vi "main 6th.vi"() -> ()   [LabVIEW 2015]
panel:
  out "6":u32
  out "3":u32
  out "1":u32
  out "2":u32
  out "5":u32
  out "4":u32
  in  "dimension size 2":i32
  in  "dimension size":i32
  out "Array":u16[][](array[numeric])
  out "element":u16[][](array[numeric])
  out "From OD fit?":bool
  in  "Current file num":i32
  in  "Fitting Results Save Path":string[](array[string])
  in  "Initial guess values":dbl[](array[numeric])
  out "Latest image data":dbl[][](array[numeric])
  in  "Fitting Type":u16(ring)
  in  "Force Guess?":bool
  in  "milliseconds to wait":u32
  out "best fit parameters":dbl[](array[numeric])
  in  "Reset process index":bool
  out "ROI Height":u32
  out "ROI Width":u32
  out "OD image":u16[][](graph)
  out "Process Index":i32
  out "External Trigger":bool
  out "XY图":cluster{i32[], dbl[]}[](graph)
  in  "OD fit":bool
  in  "OD num":i32
  out "Fit Done":bool
  in  "Exit":bool
  out "XY图 2":cluster{i32[], dbl[]}[](graph)
  in  "Fit":bool
  in  "Open File":bool
  in  "Auto Fit":bool
  in  "Stop":bool
  in  "Aquire":bool
  in  "Fitting Config":bool
  in  "Camera Config":bool
  in  "Initialize":bool
  in  "Live Image Display":refnum<k7>(container)
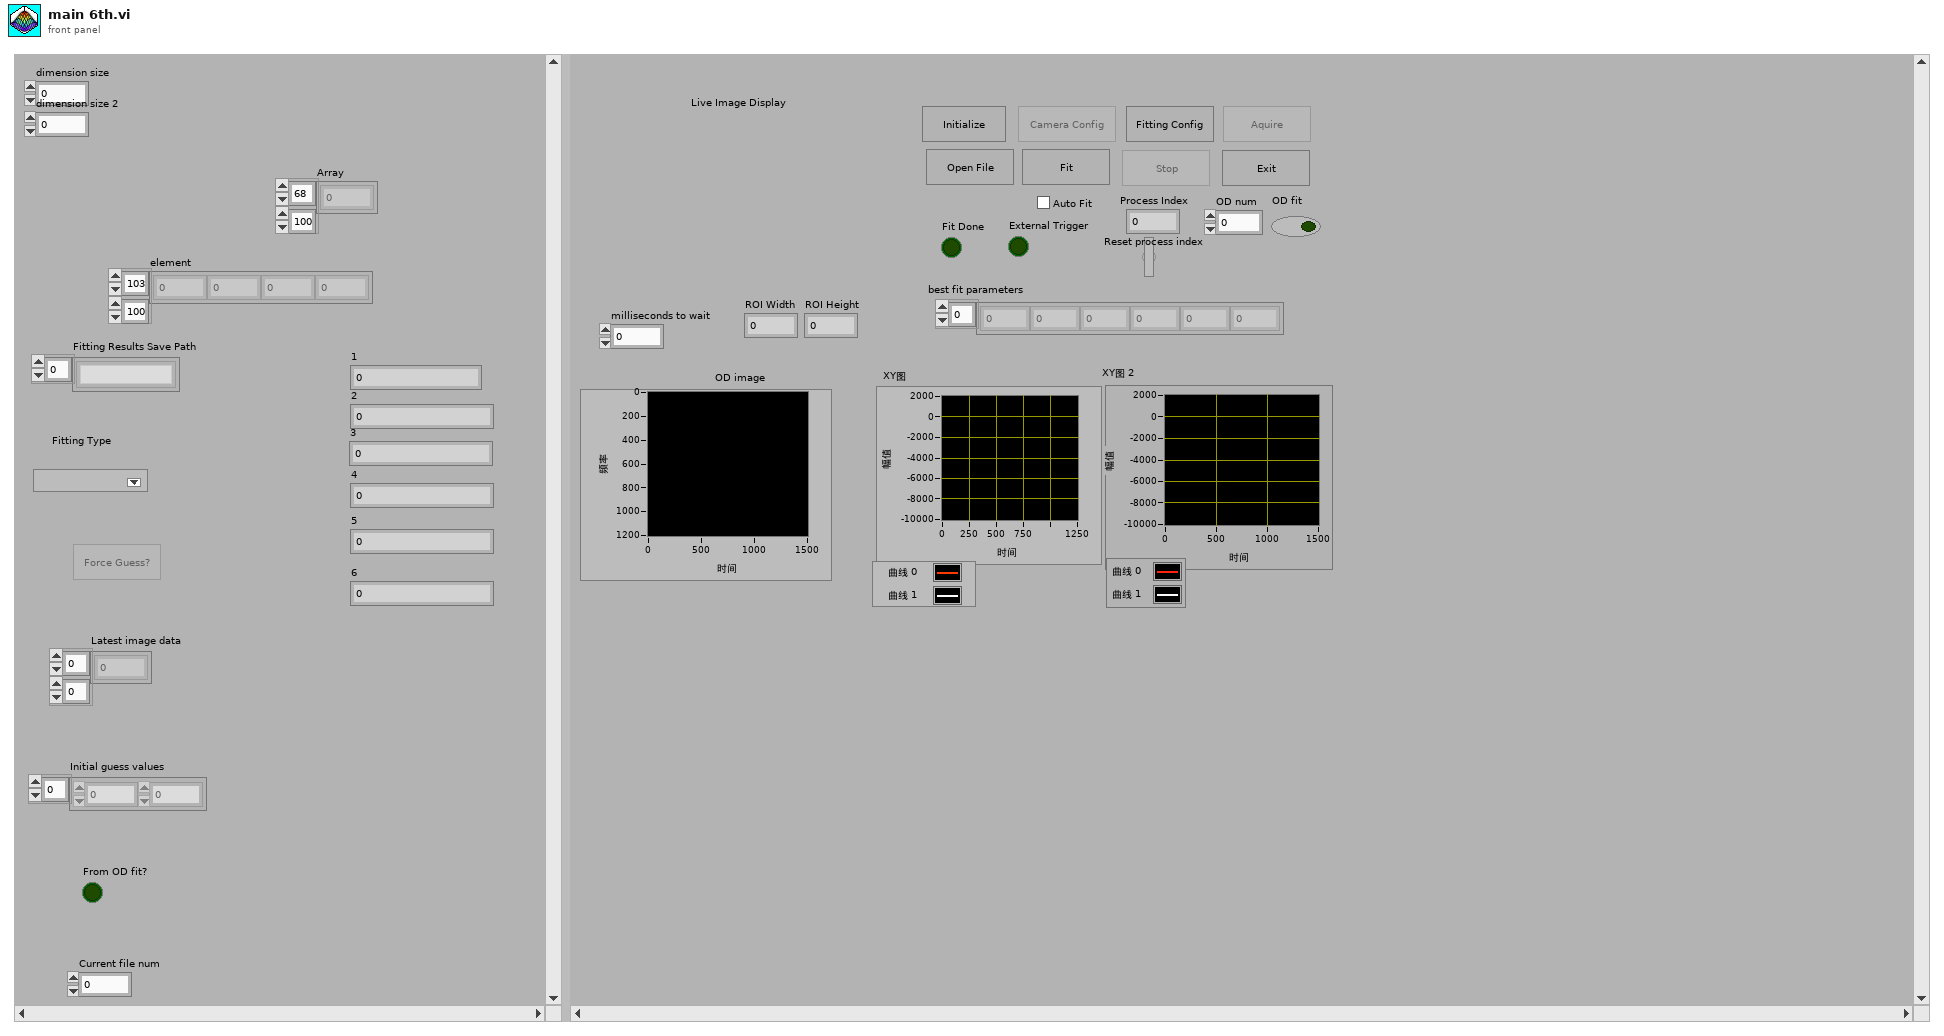
[diagram p1: front panel]
types:
  T1 = enum8{"Enabled", "Disabled", "Disabled and Grayed Out"}
  T2 = typedef "Image Type" = u32
  T3 = typedef "IMAQ Image.ctl" = refnum<image>
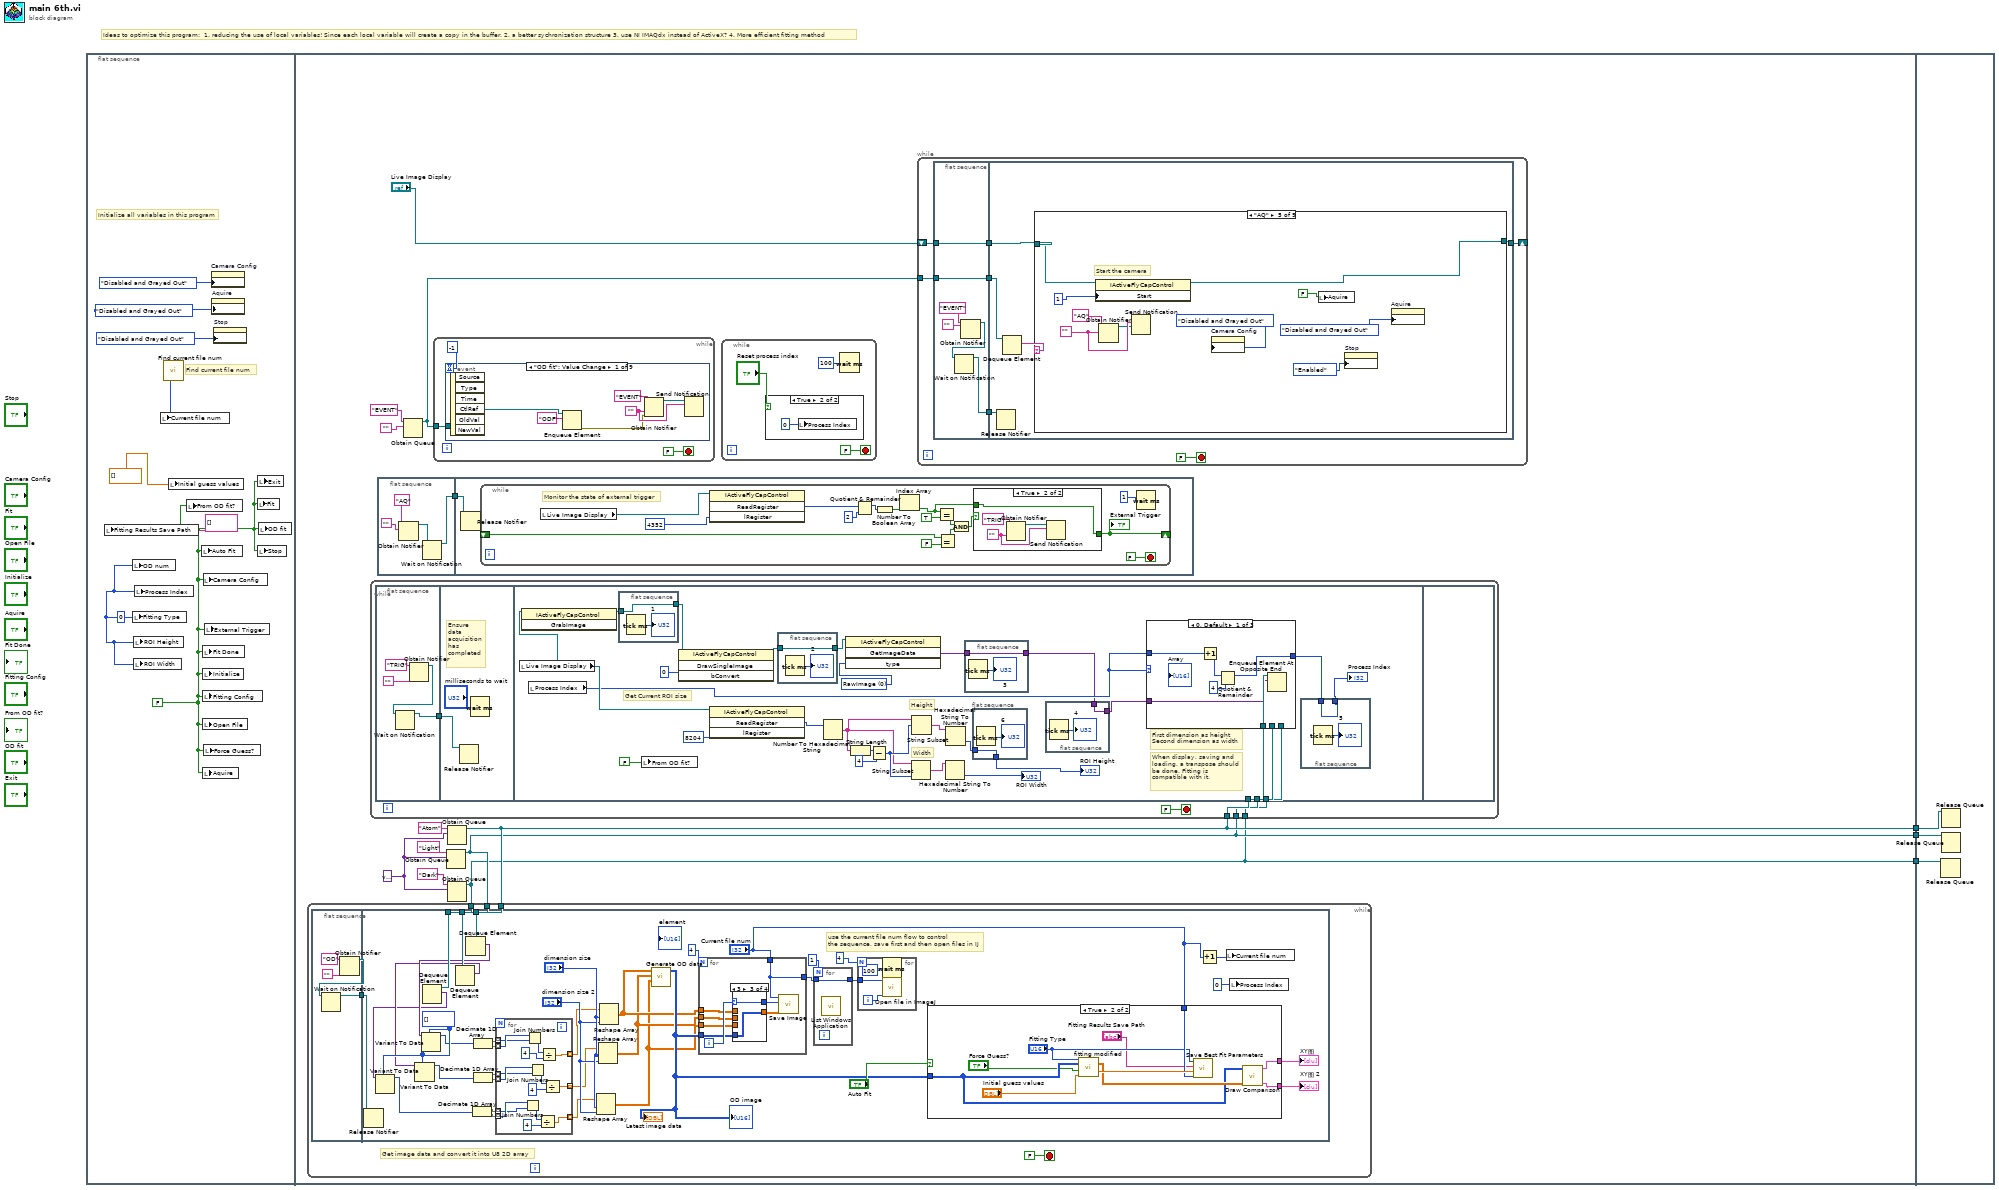
[diagram p0: block diagram]
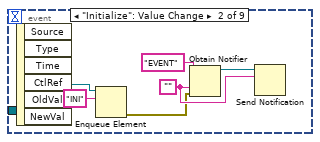
[diagram p2: hidden frame]
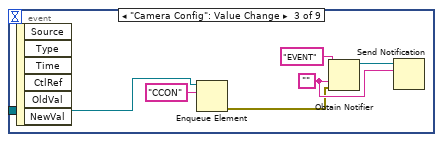
[diagram p3: hidden frame]
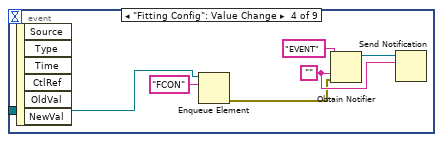
[diagram p4: hidden frame]
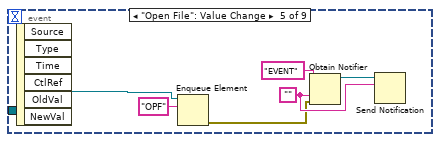
[diagram p5: hidden frame]
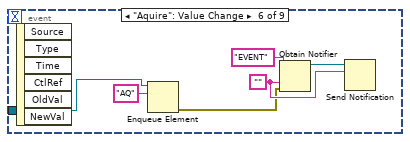
[diagram p6: hidden frame]
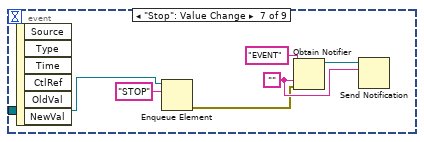
[diagram p7: hidden frame]
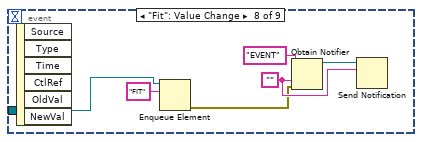
[diagram p8: hidden frame]
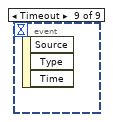
[diagram p9: hidden frame]
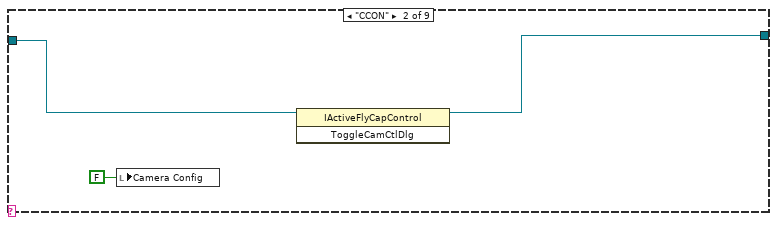
[diagram p11: hidden frame]
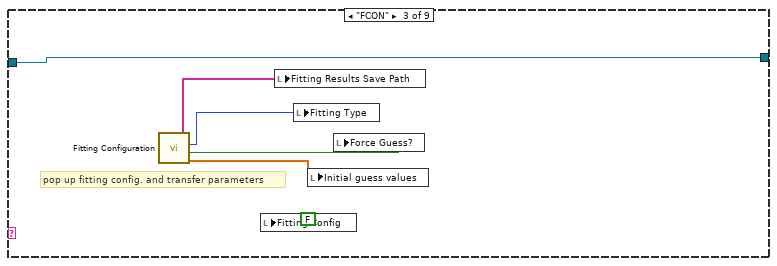
[diagram p12: hidden frame]
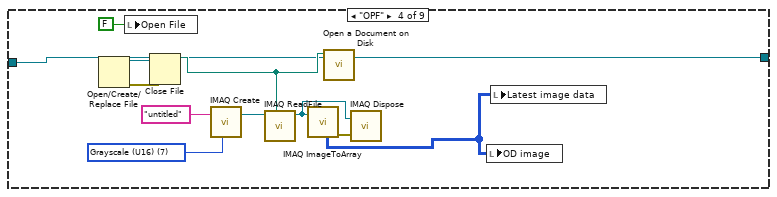
[diagram p13: hidden frame]
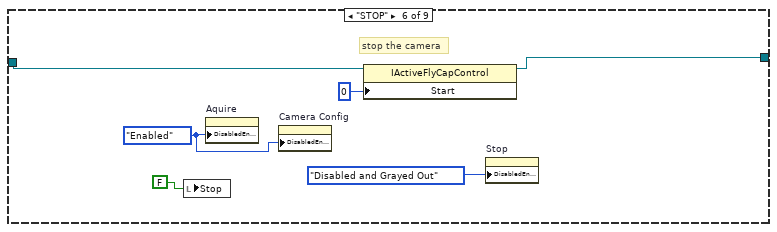
[diagram p14: hidden frame]
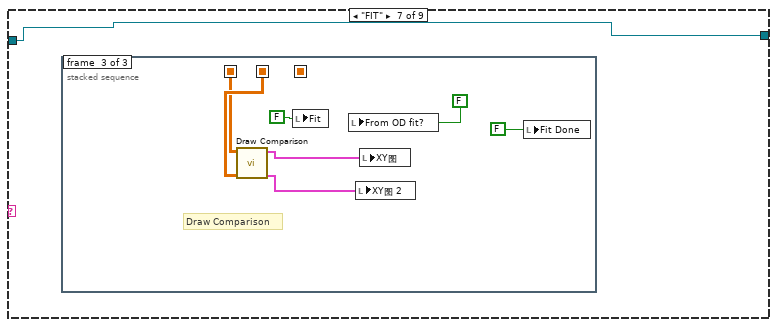
[diagram p15: hidden frame]
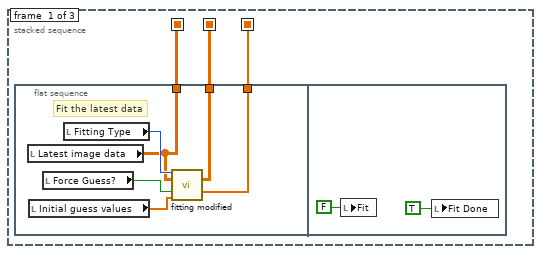
[diagram p16: hidden frame]
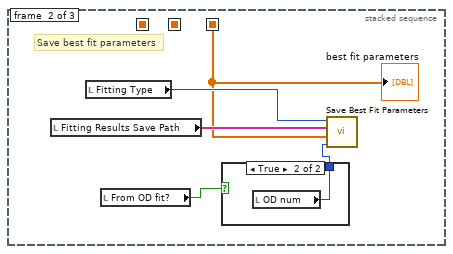
[diagram p17: hidden frame]
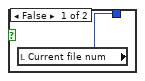
[diagram p18: hidden frame]
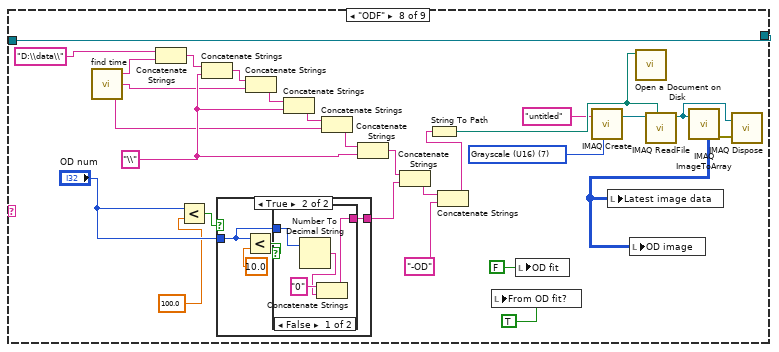
[diagram p19: hidden frame]
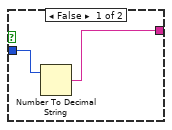
[diagram p20: hidden frame]
diagram:
  # "Ideas to optimize this program:  1. reducing the use of local variables! Since each local variable will create a copy in the buffer. 2. a better sychronization structure 3. use NI IMAQdx instead of ActiveX? 4. More efficient fitting method"
  n1 = flat-sequence {
    tunnel: [w19] -> w3
    tunnel: [w18] -> w2
    tunnel: [w17] -> w1
    tunnel: w3 -> [w411]
    tunnel: w2 -> [w410]
    tunnel: w1 -> [w409]
    frame #0 {
      w7 = 0 ("OD num")
      w5 = FALSE ("Aquire")
      # "Find current file num"
      # "Initialize all variables in this program"
      n2 = local write "Fitting Results Save Path"(string[] [] ("Fitting Results Save Path")) -> ()
      n3 = local write "OD num"(w7) -> ()
      n4 = local write "Fitting Type"(w7) -> ()
      n5 = local write "ROI Height"(w7) -> ()
      n6 = local write "ROI Width"(w7) -> ()
      n7 = local write "Process Index"(w7) -> ()
      n8 = call "Find current file num.vi"() -> ("Current File Num"=w4:u16)  [unwired: 2 in]
      n9 = local write "Current file num"(w4) -> ()
      n10 = local write "Initial guess values"(dbl[] [] ("Best fit parameters")) -> ()
      n11 = local write "From OD fit?"(w5) -> ()
      n12 = local write "Auto Fit"(w5) -> ()
      n13 = local write "Fit Done"(w5) -> ()
      n14 = local write "Initialize"(w5) -> ()
      n15 = local write "Fitting Config"(w5) -> ()
      n16 = local write "Open File"(w5) -> ()
      n17 = local write "Aquire"(w5) -> ()
      n18 = local write "Camera Config"(w5) -> ()
      n19 = local write "Force Guess?"(w5) -> ()
      n20 = local write "External Trigger"(w5) -> ()
      n21 = property on="Camera Config" class="Bool (strict)"("DisabledEnum"=T1."Disabled and Grayed Out" ("禁用")) -> ()  [unwired: 2 in, 2 out]
      n22 = property on="Aquire" class="Bool (strict)"("DisabledEnum"=T1."Disabled and Grayed Out" ("禁用")) -> ()  [unwired: 2 in, 2 out]
      n23 = property on="Stop" class="Bool (strict)"("DisabledEnum"=T1."Disabled and Grayed Out" ("禁用")) -> ()  [unwired: 2 in, 2 out]
      n24 = local write "Fit"(w5) -> ()
      n25 = local write "Exit"(w5) -> ()
      n26 = local write "Stop"(w5) -> ()
      n27 = local write "OD fit"(w5) -> ()
    }
    frame #1 {
      w13 = variant
      n28 = flat-sequence {
        tunnel: [w307] -> w23
        tunnel: w23 -> [w311]
        frame #0 {
          n29 = Obtain Notifier(name (unnamed)="AQ" ("名称（未命名）"), notification data type="") -> (notifier out=w309:refnum<notifier>)  [unwired: 2 in, 2 out]
          n30 = Wait on Notification(notifier=w309) -> (notifier out=w307:refnum<notifier>)  [unwired: 3 in, 3 out]
        }
        frame #1 {
          n31 = Release Notifier(notifier=w311) -> ()  [unwired: 2 in, 3 out]
          n32 = while {
            shift-right: [w314] -> _
            shift-left: _ -> [w313]
            stop <- FALSE stop-if-true
            # "Monitor the state of external trigger"
            n33 = local read "Live Image Display"() -> (w327:refnum<k7>)
            n34 = invoke class="IActiveFlyCapControl" method="ReadRegister"(reference=w327, "lRegister"=u32 4352) -> ("ReadRegister"=w325:u32)  [unwired: 2 in, 3 out]
            n35 = Quotient & Remainder(x=w325, y=u32 2) -> (x-y*floor(x/y)=w323:u32)  [unwired: 1 out]
            n36 = Number To Boolean Array(number=w323) -> (Boolean array=w322:bool[])
            n37 = Index Array(array=w322) -> (element=w316:bool)  [unwired: 1 in]
            n38 = Equal?(x=w316, y=TRUE) -> (x = y?=w318:bool)
            n39 = Equal?(x=w313, y=FALSE) -> (x = y?=w319:bool)
            n40 = And(x=w318, y=w319) -> (x .and. y?=w317:bool)
            n41 = case shown="True" w317 {
              tunnel: w316 -> [w328 w329]
              tunnel: [w328 w329] -> w314
              frame False {
              }
              frame True {
                w330 = ""
                n42 = Obtain Notifier(name (unnamed)="TRIG" ("名称（未命名）"), notification data type=w330) -> (notifier out=w331:refnum<notifier>)  [unwired: 2 in, 2 out]
                n43 = Send Notification(notification=w330, notifier=w331) -> ()  [unwired: 1 in, 2 out]
              }
            }
            "External Trigger" <- w314
            n44 = Wait (ms)(milliseconds to wait=u32 1) -> ()  [unwired: 1 out]
          }
        }
      }
      n45 = Obtain Queue(name (unnamed)="EVENT" ("名称（未命名）"), element data type="") -> (queue out=w14:refnum<queue>)  [unwired: 3 in, 2 out]
      n46 = while {
        tunnel: w14 -> [w24]
        stop <- FALSE stop-if-true
        n47 = event shown="[0] \"OD fit\": Value Change" {
          selector: _ -> [_ _ _ _ _ _ _ _ _]
          dyn-events: _ -> [_ _ _ _ _ _ _ _ _]
          timeout: -1 -> [_ _ _ _ _ _ _ _ _]
          tunnel: w24 -> [w27 w34 w39 w45 w51 w57 w63 w69 _]
          event "OD fit": Value Change {
            w30 = ""
            n48 = event-data() -> ()  [unwired: 1 in, 6 out]
            n49 = Enqueue Element(queue=w27, element="ODF") -> (error out=w28:errorcluster)  [unwired: 2 in, 2 out]
            n50 = Obtain Notifier(name (unnamed)="EVENT" ("名称（未命名）"), notification data type=w30, error in (no error)=w28) -> (notifier out=w31:refnum<notifier>)  [unwired: 1 in, 2 out]
            n51 = Send Notification(notification=w30, notifier=w31) -> ()  [unwired: 1 in, 2 out]
          }
          event "Initialize": Value Change {
            w36 = ""
            n52 = event-data() -> ()  [unwired: 1 in, 6 out]
            n53 = Enqueue Element(queue=w34, element="INI") -> (error out=w33:errorcluster)  [unwired: 2 in, 2 out]
            n54 = Obtain Notifier(name (unnamed)="EVENT" ("名称（未命名）"), notification data type=w36, error in (no error)=w33) -> (notifier out=w37:refnum<notifier>)  [unwired: 1 in, 2 out]
            n55 = Send Notification(notification=w36, notifier=w37) -> ()  [unwired: 1 in, 2 out]
          }
          event "Camera Config": Value Change {
            w42 = ""
            n56 = event-data() -> ()  [unwired: 1 in, 6 out]
            n57 = Enqueue Element(queue=w39, element="CCON") -> (error out=w40:errorcluster)  [unwired: 2 in, 2 out]
            n58 = Obtain Notifier(name (unnamed)="EVENT" ("名称（未命名）"), notification data type=w42, error in (no error)=w40) -> (notifier out=w43:refnum<notifier>)  [unwired: 1 in, 2 out]
            n59 = Send Notification(notification=w42, notifier=w43) -> ()  [unwired: 1 in, 2 out]
          }
          event "Fitting Config": Value Change {
            w48 = ""
            n60 = event-data() -> ()  [unwired: 1 in, 6 out]
            n61 = Enqueue Element(queue=w45, element="FCON") -> (error out=w46:errorcluster)  [unwired: 2 in, 2 out]
            n62 = Obtain Notifier(name (unnamed)="EVENT" ("名称（未命名）"), notification data type=w48, error in (no error)=w46) -> (notifier out=w49:refnum<notifier>)  [unwired: 1 in, 2 out]
            n63 = Send Notification(notification=w48, notifier=w49) -> ()  [unwired: 1 in, 2 out]
          }
          event "Open File": Value Change {
            w54 = ""
            n64 = event-data() -> ()  [unwired: 1 in, 6 out]
            n65 = Enqueue Element(queue=w51, element="OPF") -> (error out=w52:errorcluster)  [unwired: 2 in, 2 out]
            n66 = Obtain Notifier(name (unnamed)="EVENT" ("名称（未命名）"), notification data type=w54, error in (no error)=w52) -> (notifier out=w55:refnum<notifier>)  [unwired: 1 in, 2 out]
            n67 = Send Notification(notification=w54, notifier=w55) -> ()  [unwired: 1 in, 2 out]
          }
          event "Aquire": Value Change {
            w60 = ""
            n68 = event-data() -> ()  [unwired: 1 in, 6 out]
            n69 = Enqueue Element(queue=w57, element="AQ") -> (error out=w58:errorcluster)  [unwired: 2 in, 2 out]
            n70 = Obtain Notifier(name (unnamed)="EVENT" ("名称（未命名）"), notification data type=w60, error in (no error)=w58) -> (notifier out=w61:refnum<notifier>)  [unwired: 1 in, 2 out]
            n71 = Send Notification(notification=w60, notifier=w61) -> ()  [unwired: 1 in, 2 out]
          }
          event "Stop": Value Change {
            w66 = ""
            n72 = event-data() -> ()  [unwired: 1 in, 6 out]
            n73 = Enqueue Element(queue=w63, element="STOP") -> (error out=w64:errorcluster)  [unwired: 2 in, 2 out]
            n74 = Obtain Notifier(name (unnamed)="EVENT" ("名称（未命名）"), notification data type=w66, error in (no error)=w64) -> (notifier out=w67:refnum<notifier>)  [unwired: 1 in, 2 out]
            n75 = Send Notification(notification=w66, notifier=w67) -> ()  [unwired: 1 in, 2 out]
          }
          event "Fit": Value Change {
            w72 = ""
            n76 = event-data() -> ()  [unwired: 1 in, 6 out]
            n77 = Enqueue Element(queue=w69, element="FIT") -> (error out=w70:errorcluster)  [unwired: 2 in, 2 out]
            n78 = Obtain Notifier(name (unnamed)="EVENT" ("名称（未命名）"), notification data type=w72, error in (no error)=w70) -> (notifier out=w73:refnum<notifier>)  [unwired: 1 in, 2 out]
            n79 = Send Notification(notification=w72, notifier=w73) -> ()  [unwired: 1 in, 2 out]
          }
          event Timeout {
            n80 = event-data() -> ()  [unwired: 1 in, 3 out]
          }
        }
      }
      n81 = Obtain Queue(name (unnamed)="Light" ("名称（未命名）"), element data type=w13) -> (queue out=w18:refnum<queue>)  [unwired: 3 in, 2 out]
      n82 = Obtain Queue(name (unnamed)="Atom" ("名称（未命名）"), element data type=w13) -> (queue out=w19:refnum<queue>)  [unwired: 3 in, 2 out]
      n83 = Obtain Queue(name (unnamed)="Dark" ("名称（未命名）"), element data type=w13) -> (queue out=w17:refnum<queue>)  [unwired: 3 in, 2 out]
      n84 = while {
        tunnel: w19 -> [w216]
        tunnel: w18 -> [w215]
        tunnel: w17 -> [w214]
        stop <- FALSE stop-if-true
        # "Get image data and convert it into U8 2D array"
        n85 = flat-sequence {
          tunnel: [w218] -> w217
          tunnel: w217 -> [w225]
          tunnel: w216 -> [w257]
          tunnel: w215 -> [w256]
          tunnel: w214 -> [w255]
          frame #0 {
            n86 = Obtain Notifier(name (unnamed)="OD" ("名称（未命名）"), notification data type="") -> (notifier out=w219:refnum<notifier>)  [unwired: 2 in, 2 out]
            n87 = Wait on Notification(notifier=w219) -> (notifier out=w218:refnum<notifier>)  [unwired: 3 in, 3 out]
          }
          frame #1 {
            w228 = u8[] []
            # "use the current file num flow to control \nthe sequence, save first and then open files in IJ"
            n88 = Release Notifier(notifier=w225) -> ()  [unwired: 2 in, 3 out]
            n89 = Dequeue Element(queue=w255) -> (element=w226:variant)  [unwired: 2 in, 3 out]
            n90 = Variant To Data(type=w228, Variant=w226) -> (data=w222:u8[])  [unwired: 1 in, 1 out]
            n91 = Dequeue Element(queue=w256) -> (element=w227:variant)  [unwired: 2 in, 3 out]
            n92 = Variant To Data(type=w228, Variant=w227) -> (data=w223:u8[])  [unwired: 1 in, 1 out]
            n93 = Dequeue Element(queue=w257) -> (element=w229:variant)  [unwired: 2 in, 3 out]
            n94 = Variant To Data(type=w228, Variant=w229) -> (data=w224:u8[])  [unwired: 1 in, 1 out]
            n95 = Decimate 1D Array(w222) -> (w239:u8[], w238:u8[])
            n96 = Decimate 1D Array(w224) -> (w243:u8[], w242:u8[])
            n97 = Decimate 1D Array(w223) -> (w241:u8[], w240:u8[])
            n98 = for {
              tunnel: [w271] -> w235 mode=indexing
              tunnel: w243 -> [w261] mode=indexing
              tunnel: w242 -> [w262] mode=indexing
              tunnel: w241 -> [w263] mode=indexing
              tunnel: w240 -> [w264] mode=indexing
              tunnel: w239 -> [w265] mode=indexing
              tunnel: w238 -> [w266] mode=indexing
              tunnel: [w260] -> w234 mode=indexing
              tunnel: [w259] -> w233 mode=indexing
              n99 = Join Numbers(hi=w266, lo=w265) -> ((hi.lo)=w268:u16)
              n100 = Join Numbers(hi=w262, lo=w261) -> ((hi.lo)=w273:u16)
              n101 = Join Numbers(hi=w264, lo=w263) -> ((hi.lo)=w270:u16)
              n102 = Divide(x=w268, y=u16 4) -> (x/y=w259:dbl)
              n103 = Divide(x=w273, y=u16 4) -> (x/y=w271:dbl)
              n104 = Divide(x=w270, y=u16 4) -> (x/y=w260:dbl)
            }
            n105 = Reshape Array(w233, "dimension size", "dimension size 2") -> (w230:dbl[][])
            n106 = Reshape Array(w234, "dimension size", "dimension size 2") -> (w231:dbl[][])
            n107 = Reshape Array(w235, "dimension size", "dimension size 2") -> (w232:dbl[][])
            n108 = call "Generate OD data.vi"("dark"=w230, "light"=w231, "atom"=w232) -> ("OD image"=w251:u16[][])  [unwired: 3 in]
            "OD image" <- w251
            "Latest image data" <- w251
            n109 = for {
              N: 4 -> [_]
              tunnel: w232 -> [w297]
              tunnel: w231 -> [w296]
              tunnel: w230 -> [w295]
              tunnel: w251 -> [w294]
              tunnel: "Current file num" -> [w291]
              tunnel: [w291] -> w244
              i -> [w298]
              n110 = case shown="3" w298 {
                selector: w298 -> [w300 w302 w304 w306]
                tunnel: w297 -> [w299 _ _ _]
                tunnel: w296 -> [_ _ _ w305]
                tunnel: w295 -> [_ w301 _ _]
                tunnel: w294 -> [_ _ w303 _]
                tunnel: [w300 w302 w304 w306] -> w293
                tunnel: [w299 w301 w303 w305] -> w292
                frame 0, Default {
                }
                frame 2 {
                }
                frame 3 {
                }
                frame 1 {
                }
              }
              n111 = call "Save Image.vi"("Data"=w292, "Process Index"=w293, "Current File Num"=w291) -> ()  [unwired: 9 in]
            }
            n112 = for {
              N: 1 -> [_]
              tunnel: w244 -> [w274]
              tunnel: [w274] -> w246
              n113 = call "List Windows Application.vi"() -> ()  [unwired: 1 in]
            }
            n114 = for {
              N: 4 -> [_]
              tunnel: w246 -> [w277]
              i -> [w276]
              n115 = Wait (ms)(milliseconds to wait=u32 100) -> ()  [unwired: 1 out]
              n116 = call "Open file in ImageJ.vi"("Process Index"=w276, "Current File Num"=w277) -> ()  [unwired: 10 in]
            }
            n117 = case shown="True" "Auto Fit" {
              tunnel: w251 -> [w280 w287]
              tunnel: "Current file num" -> [_ w289]
              tunnel: [w279 w286] -> w252
              tunnel: [w278 w285] -> w253
              frame False {
                n118 = call "Draw Comparison.vi"("Best Fit"=w280, "Raw Data"=w280) -> ("Vertical Comparison"=w278:cluster{i32[], dbl[]}[], "Horizontal Comparison"=w279:cluster{i32[], dbl[]}[])  [unwired: 7 in]
              }
              frame True {
                n119 = call "fitting modified.vi"("fitting type"="Fitting Type", "2D data"=w287, "force guess?"="Force Guess?", "intial guess value"="Initial guess values") -> ("best fit"=w288:dbl[][], "best fit parameters"=w290:dbl[])  [unwired: 8 in, 2 out]
                n120 = call "Save Best Fit Parameters.vi"("Current File Num"=w289, "Best Fit Parameters"=w290, "Fitting Results Save Path"="Fitting Results Save Path", "Fitting Type"="Fitting Type") -> ()  [unwired: 8 in]
                n121 = call "Draw Comparison.vi"("Best Fit"=w288, "Raw Data"=w287) -> ("Vertical Comparison"=w285:cluster{i32[], dbl[]}[], "Horizontal Comparison"=w286:cluster{i32[], dbl[]}[])  [unwired: 7 in]
              }
            }
            "XY图" <- w252
            "XY图 2" <- w253
            n122 = Increment(x="Current file num") -> (x+1=w250:i32)
            n123 = local write "Current file num"(w250) -> ()
            n124 = local write "Process Index"(0 ("Process Index")) -> ()
          }
        }
      }
      n125 = while {
        tunnel: w19 -> [w336]
        tunnel: w18 -> [w335]
        tunnel: w17 -> [w334]
        stop <- FALSE stop-if-true
        n126 = flat-sequence {
          tunnel: [w338] -> w337
          tunnel: w337 -> [w343]
          tunnel: w336 -> [w359]
          tunnel: w335 -> [w358]
          tunnel: w334 -> [w357]
          frame #0 {
            n127 = Obtain Notifier(name (unnamed)="TRIG" ("名称（未命名）"), notification data type="") -> (notifier out=w339:refnum<notifier>)  [unwired: 2 in, 2 out]
            n128 = Wait on Notification(notifier=w339) -> (notifier out=w338:refnum<notifier>)  [unwired: 3 in, 3 out]
          }
          frame #1 {
            # "Ensure\ndata\nacquisition\nhas \ncompleted"
            n129 = Release Notifier(notifier=w343) -> ()  [unwired: 2 in, 3 out]
            n130 = Wait (ms)(milliseconds to wait="milliseconds to wait") -> ()  [unwired: 1 out]
          }
          frame #2 {
            w371 = 0 items=["RawImage", "ColorProcessedImage"] ("type")
            # "When display, saving and \nloading, a transpose should\nbe done. Fitting is \ncompatible with it."
            # "First dimension as height\nSecond dimension as width"
            # "Width"
            # "Height"
            # "Get Current ROI size"
            n131 = local read "Live Image Display"() -> (w361:refnum<k7>)
            n132 = invoke class="IActiveFlyCapControl" method="GrabImage"(reference=w361) -> (reference out=w348:refnum<k7>)  [unwired: 2 in, 2 out]
            n133 = local read "Process Index"() -> (w360:i32)
            n134 = flat-sequence {
              tunnel: [w376] -> w349
              tunnel: w348 -> [w376]
              frame #0 {
                n135 = Tick Count (ms)() -> (millisecond timer value=→"1":u32)
              }
            }
            n136 = local write "From OD fit?"(FALSE ("From OD fit?")) -> ()
            n137 = invoke class="IActiveFlyCapControl" method="DrawSingleImage"(reference=w349, "bConvert"=0) -> (reference out=w351:refnum<k7>)  [unwired: 2 in, 3 out]
            n138 = invoke class="IActiveFlyCapControl" method="ReadRegister"(reference=w361, "lRegister"=u32 8204) -> ("ReadRegister"=w369:u32)  [unwired: 2 in, 3 out]
            n139 = flat-sequence {
              tunnel: w351 -> [w378]
              tunnel: [w378] -> w350
              frame #0 {
                n140 = Tick Count (ms)() -> (millisecond timer value=→"2":u32)
              }
            }
            n141 = Number To Hexadecimal String(2:w369) -> (0:w365:string)  [unwired: 1 in]
            n142 = invoke class="IActiveFlyCapControl" method="GetImageData"(reference=w350, "type"=w371) -> ("GetImageData"=w347:variant)  [unwired: 2 in, 3 out]
            n143 = String Length(string=w365) -> (length=w368:i32)
            n144 = Subtract(x=w368, y=4) -> (x-y=w366:i32)
            n145 = String Subset(string=w365, length (rest)=w366) -> (substring=w363:string)  [unwired: 1 in]
            n146 = String Subset(string=w365, offset (0)=w366) -> (substring=w364:string)  [unwired: 1 in]
            n147 = Hexadecimal String To Number(string=w363) -> (number=→"ROI Width":u32)  [unwired: 2 in, 1 out]
            n148 = Hexadecimal String To Number(string=w364) -> (number=w345:u32)  [unwired: 2 in, 1 out]
            n149 = flat-sequence {
              tunnel: [w374] -> w344
              tunnel: w347 -> [w374]
              frame #0 {
                n150 = Tick Count (ms)() -> (millisecond timer value=→"3":u32)
              }
            }
            n151 = flat-sequence {
              tunnel: [w372] -> w346
              tunnel: w345 -> [w372]
              frame #0 {
                n152 = Tick Count (ms)() -> (millisecond timer value=→"6":u32)
              }
            }
            n153 = flat-sequence {
              tunnel: w344 -> [w383]
              tunnel: [w383] -> w352
              frame #0 {
                n154 = Tick Count (ms)() -> (millisecond timer value=→"4":u32)
              }
            }
            n155 = case shown="0, Default" w360 {
              tunnel: w360 -> [w387 w393 w399]
              tunnel: w352 -> [w384 w390 w398]
              tunnel: w359 -> [w385 _ _]
              tunnel: w358 -> [_ w391 _]
              tunnel: w357 -> [_ _ w397]
              tunnel: [w386 w392 w396] -> w354
              frame 0, Default {
                n156 = Increment(x=w387) -> (x+1=w388:i32)
                n157 = Quotient & Remainder(x=w388, y=4) -> (x-y*floor(x/y)=w386:i32)  [unwired: 1 out]
                n158 = Enqueue Element At Opposite End(queue=w385, element=w384) -> ()  [unwired: 2 in, 3 out]
              }
              frame 1 {
                n159 = Increment(x=w393) -> (x+1=w394:i32)
                n160 = Quotient & Remainder(x=w394, y=4) -> (x-y*floor(x/y)=w392:i32)  [unwired: 1 out]
                n161 = Enqueue Element At Opposite End(queue=w391, element=w390) -> ()  [unwired: 2 in, 3 out]
              }
              frame 2 {
                n162 = stacked-sequence {
                  tunnel: w399 -> [w403 _]
                  tunnel: w398 -> [w400 _]
                  tunnel: w397 -> [w401 _]
                  tunnel: [w402 _] -> w396
                  frame #0 {
                    n163 = Increment(x=w403) -> (x+1=w404:i32)
                    n164 = Quotient & Remainder(x=w404, y=4) -> (x-y*floor(x/y)=w402:i32)  [unwired: 1 out]
                    n165 = Enqueue Element At Opposite End(queue=w401, element=w400) -> ()  [unwired: 2 in, 3 out]
                  }
                  frame #1 {
                    w406 = ""
                    n166 = Obtain Notifier(name (unnamed)="OD" ("名称（未命名）"), notification data type=w406) -> (notifier out=w408:refnum<notifier>)  [unwired: 2 in, 2 out]
                    n167 = Send Notification(notification=w406, notifier=w408) -> ()  [unwired: 1 in, 2 out]
                  }
                }
              }
            }
            n168 = flat-sequence {
              tunnel: w354 -> [w381]
              tunnel: [w381] -> w353
              frame #0 {
                n169 = Tick Count (ms)() -> (millisecond timer value=→"5":u32)
              }
            }
            "ROI Height" <- w346
            "Process Index" <- w353
          }
          frame #3 {
          }
        }
      }
      n170 = while {
        stop <- FALSE stop-if-true
        n171 = case shown="True" "Reset process index" {
          frame False {
          }
          frame True {
            n172 = local write "Process Index"(0 ("Process Index")) -> ()
          }
        }
        n173 = Wait (ms)(milliseconds to wait=u32 100 ("等待时间（毫秒）")) -> ()  [unwired: 1 out]
      }
      n174 = while {
        tunnel: w14 -> [w79]
        shift-right: [w75] -> _
        shift-left: "Live Image Display" -> [w76]
        stop <- FALSE stop-if-true
        n175 = flat-sequence {
          tunnel: [w84] -> w81
          tunnel: w79 -> [w83]
          tunnel: [w83] -> w78
          tunnel: [w82] -> w77
          tunnel: w76 -> [w82]
          tunnel: w81 -> [w92]
          tunnel: w78 -> [w91]
          tunnel: w77 -> [w89]
          tunnel: [w88] -> w75
          frame #0 {
            n176 = Obtain Notifier(name (unnamed)="EVENT" ("名称（未命名）"), notification data type="") -> (notifier out=w85:refnum<notifier>)  [unwired: 2 in, 2 out]
            n177 = Wait on Notification(notifier=w85) -> (notifier out=w84:refnum<notifier>)  [unwired: 3 in, 3 out]
          }
          frame #1 {
            n178 = Release Notifier(notifier=w92) -> ()  [unwired: 2 in, 3 out]
            n179 = Dequeue Element(queue=w91) -> (element=w90:string)  [unwired: 2 in, 3 out]
            n180 = case shown="\"AQ\"" w90 {
              tunnel: w89 -> [w93 w95 w97 w103 w115 w125 w130 w156 w198]
              tunnel: [w93 w94 w97 w103 w114 w124 w130 w156 w199] -> w88
              frame Default {
              }
              frame "CCON" {
                n181 = local write "Camera Config"(FALSE ("Camera Config")) -> ()
                n182 = invoke class="IActiveFlyCapControl" method="ToggleCamCtlDlg"(reference=w95) -> (reference out=w94:refnum<k7>)  [unwired: 2 in, 2 out]
              }
              frame "FCON" {
                # "pop up fitting config. and transfer parameters"
                n183 = call "Fitting Configuration.vi"() -> ("intial guess"=w102:dbl[], "Force Guess？"=w101:bool, "Fitting Type"=w99:u16, "Fitting Results Save Path"=w100:string[])  [unwired: 5 in]
                n184 = local write "Fitting Config"(FALSE ("Fitting Config")) -> ()
                n185 = local write "Fitting Results Save Path"(w100) -> ()
                n186 = local write "Fitting Type"(w99) -> ()
                n187 = local write "Initial guess values"(w102) -> ()
                n188 = local write "Force Guess?"(w101) -> ()
              }
              frame "OPF" {
                w105 = T2 7 items=["Grayscale (U8)", "Grayscale (I16)", "Grayscale (SGL)", "Complex (CSG)", "RGB (U32)", "HSL (U32)", "RGB (U64)", "Grayscale (U16)"] ("Image Type")
                n189 = Open/Create/Replace File() -> (refnum out=w112:refnum<file>, error out=w111:errorcluster)  [unwired: 6 in, 1 out]
                n190 = local write "Open File"(FALSE ("Open File")) -> ()
                n191 = Close File(refnum=w112, error in=w111) -> (path=w113:path)  [unwired: 1 out]
                n192 = call "IMAQ Create"("Image Name"="untitled", "Image Type"=w105) -> ("New Image"=w106:T3)  [unwired: 3 in, 1 out]
                n193 = call "IMAQ ReadFile"("File Path"=w113, "Image"=w106) -> ("Image Out"=w107:T3)  [unwired: 5 in, 4 out]
                n194 = call "IMAQ ImageToArray"("Image"=w107) -> ("Image Pixels (U16)"=w110:u16[][], "error out"=w108:errorcluster)  [unwired: 3 in, 3 out]
                n195 = call <vilib>:"Open a Document on Disk.vi"("document path"=w113) -> ()  [unwired: 6 in, 1 out]
                n196 = call "IMAQ Dispose"("Image"=w107, "error in (no error)"=w108) -> ()  [unwired: 4 in, 1 out]
                n197 = local write "OD image"(w110) -> ()
                n198 = local write "Latest image data"(w110) -> ()
              }
              frame "AQ" {
                w122 = ""
                # "Start the camera"
                n199 = property class="IActiveFlyCapControl"(reference=w115, "Start"=1) -> (reference out=w114:refnum<k7>)  [unwired: 1 in, 1 out]
                n200 = Obtain Notifier(name (unnamed)="AQ" ("名称（未命名）"), notification data type=w122) -> (notifier out=w121:refnum<notifier>)  [unwired: 2 in, 2 out]
                n201 = Send Notification(notification=w122, notifier=w121) -> ()  [unwired: 1 in, 2 out]
                n202 = property on="Camera Config" class="Bool (strict)"("DisabledEnum"=T1."Disabled and Grayed Out" ("禁用")) -> ()  [unwired: 2 in, 2 out]
                n203 = local write "Aquire"(FALSE ("Initialize")) -> ()
                n204 = property on="Stop" class="Bool (strict)"("DisabledEnum"=T1."Enabled" ("禁用")) -> ()  [unwired: 2 in, 2 out]
                n205 = property on="Aquire" class="Bool (strict)"("DisabledEnum"=T1."Disabled and Grayed Out" ("禁用")) -> ()  [unwired: 2 in, 2 out]
              }
              frame "STOP" {
                w129 = T1."Enabled" ("禁用")
                # "stop the camera"
                n206 = local write "Stop"(FALSE ("Initialize")) -> ()
                n207 = property on="Aquire" class="Bool (strict)"("DisabledEnum"=w129) -> ()  [unwired: 2 in, 2 out]
                n208 = property on="Camera Config" class="Bool (strict)"("DisabledEnum"=w129) -> ()  [unwired: 2 in, 2 out]
                n209 = property class="IActiveFlyCapControl"(reference=w125, "Start"=0) -> (reference out=w124:refnum<k7>)  [unwired: 1 in, 1 out]
                n210 = property on="Stop" class="Bool (strict)"("DisabledEnum"=T1."Disabled and Grayed Out" ("禁用")) -> ()  [unwired: 2 in, 2 out]
              }
              frame "FIT" {
                n211 = stacked-sequence {
                  seq-local: [w132 _ _] -> [_ _ w152]
                  seq-local: [w133 _ _] -> [_ _ w150]
                  seq-local: [w131 _ _] -> [_ w142 _]
                  frame #0 {
                    n212 = flat-sequence {
                      tunnel: [w136] -> w133
                      tunnel: [w135] -> w132
                      tunnel: [w134] -> w131
                      frame #0 {
                        # "Fit the latest data"
                        n213 = local read "Latest image data"() -> (w136:dbl[][])
                        n214 = local read "Initial guess values"() -> (w138:dbl[])
                        n215 = local read "Force Guess?"() -> (w139:bool)
                        n216 = local read "Fitting Type"() -> (w137:u16)
                        n217 = call "fitting modified.vi"("fitting type"=w137, "2D data"=w136, "force guess?"=w139, "intial guess value"=w138) -> ("best fit"=w135:dbl[][], "best fit parameters"=w134:dbl[])  [unwired: 8 in, 2 out]
                      }
                      frame #1 {
                        n218 = local write "Fit"(FALSE ("Fit")) -> ()
                        n219 = local write "Fit Done"(TRUE ("Fit Done")) -> ()
                      }
                    }
                  }
                  frame #1 {
                    # "Save best fit parameters"
                    n220 = local read "Fitting Results Save Path"() -> (w145:string[])
                    n221 = local read "Fitting Type"() -> (w146:u16)
                    n222 = local read "From OD fit?"() -> (w144:bool)
                    n223 = case shown="True" w144 {
                      tunnel: [w147 w148] -> w143
                      frame False {
                        n224 = local read "Current file num"() -> (w147:i32)
                      }
                      frame True {
                        n225 = local read "OD num"() -> (w148:i32)
                      }
                    }
                    n226 = call "Save Best Fit Parameters.vi"("Current File Num"=w143, "Best Fit Parameters"=w142, "Fitting Results Save Path"=w145, "Fitting Type"=w146) -> ()  [unwired: 8 in]
                    "best fit parameters" <- w142
                  }
                  frame #2 {
                    # "Draw Comparison"
                    n227 = call "Draw Comparison.vi"("Best Fit"=w152, "Raw Data"=w150) -> ("Vertical Comparison"=w154:cluster{i32[], dbl[]}[], "Horizontal Comparison"=w155:cluster{i32[], dbl[]}[])  [unwired: 7 in]
                    n228 = local write "Fit"(FALSE ("Initialize")) -> ()
                    n229 = local write "From OD fit?"(FALSE ("From OD fit?")) -> ()
                    n230 = local write "XY图 2"(w154) -> ()
                    n231 = local write "XY图"(w155) -> ()
                    n232 = local write "Fit Done"(FALSE ("Fit Done")) -> ()
                  }
                }
              }
              frame "ODF" {
                w177 = T2 7 items=["Grayscale (U8)", "Grayscale (I16)", "Grayscale (SGL)", "Complex (CSG)", "RGB (U32)", "HSL (U32)", "RGB (U64)", "Grayscale (U16)"] ("Image Type")
                w168 = "\\" ("字符串")
                n233 = call "find time.vi"() -> ("day"=w166:string, "month"=w163:string, "year"=w160:string)  [unwired: 3 in]
                n234 = Concatenate Strings("D:\\data\\", w160) -> (w161:string)
                n235 = Less?(x="OD num", y=100.0) -> (x < y?=w174:bool)
                n236 = Concatenate Strings(w161, w168) -> (w162:string)
                n237 = case shown="True" w174 {
                  tunnel: "OD num" -> [w185 w187]
                  tunnel: [w184 w186] -> w175
                  frame False {
                    n238 = Number To Decimal String(number=w185) -> (decimal integer string=w184:string)  [unwired: 1 in]
                  }
                  frame True {
                    n239 = Less?(x=w187, y=10.0) -> (x < y?=w188:bool)
                    n240 = case shown="False" w188 {
                      tunnel: w187 -> [w192 w197]
                      tunnel: [w190 w194] -> w186
                      frame False {
                        n241 = Number To Decimal String(number=w192) -> (decimal integer string=w191:string)  [unwired: 1 in]
                        n242 = Concatenate Strings("0" ("字符串"), w191) -> (w190:string)
                      }
                      frame True {
                        n243 = Number To Decimal String(number=w197) -> (decimal integer string=w195:string)  [unwired: 1 in]
                        n244 = Concatenate Strings("00" ("字符串"), w195) -> (w194:string)
                      }
                    }
                  }
                }
                n245 = Concatenate Strings(w162, w163) -> (w164:string)
                n246 = Concatenate Strings(w164, w168) -> (w165:string)
                n247 = Concatenate Strings(w165, w166) -> (w167:string)
                n248 = Concatenate Strings(w167, w168) -> (w169:string)
                n249 = Concatenate Strings(w169, w175) -> (w170:string)
                n250 = Concatenate Strings(w170, "-OD" ("字符串")) -> (w172:string)
                n251 = String To Path(string=w172) -> (path=w181:path)
                n252 = local write "From OD fit?"(TRUE ("From OD fit?")) -> ()
                n253 = local write "OD fit"(FALSE ("OD fit")) -> ()
                n254 = call "IMAQ Create"("Image Name"="untitled", "Image Type"=w177) -> ("New Image"=w182:T3)  [unwired: 3 in, 1 out]
                n255 = call <vilib>:"Open a Document on Disk.vi"("document path"=w181) -> ()  [unwired: 6 in, 1 out]
                n256 = call "IMAQ ReadFile"("File Path"=w181, "Image"=w182) -> ("Image Out"=w183:T3)  [unwired: 5 in, 4 out]
                n257 = call "IMAQ ImageToArray"("Image"=w183) -> ("Image Pixels (U16)"=w179:u16[][], "error out"=w178:errorcluster)  [unwired: 3 in, 3 out]
                n258 = local write "Latest image data"(w179) -> ()
                n259 = local write "OD image"(w179) -> ()
                n260 = call "IMAQ Dispose"("Image"=w183, "error in (no error)"=w178) -> ()  [unwired: 4 in, 1 out]
              }
              frame "INI" {
                w202 = 2 items=["FreeRunning", "LockNext", "LockLatest"] ("mode")
                # "Setup Camera Index"
                # "Set grab mode"
                # "Make Sure the camera is not running"
                n261 = property class="IActiveFlyCapControl"(reference=w198, "Camera"=0 ("Start")) -> (reference out=w203:refnum<k7>)  [unwired: 1 in, 1 out]
                n262 = invoke class="IActiveFlyCapControl" method="ShowCamSlnModal"(reference=w203) -> (reference out=w206:refnum<k7>)  [unwired: 2 in, 2 out]
                n263 = property class="IActiveFlyCapControl"(reference=w206, "Start"=0 ("Camera")) -> (reference out=w207:refnum<k7>)  [unwired: 1 in, 1 out]
                n264 = invoke class="IActiveFlyCapControl" method="SetGrabMode"(reference=w207, "mode"=w202) -> (reference out=w199:refnum<k7>)  [unwired: 2 in, 3 out]
                n265 = local write "Initialize"(FALSE ("Initialize")) -> ()
                n266 = property on="Camera Config" class="Bool (strict)"("DisabledEnum"=T1."Enabled" ("禁用")) -> ()  [unwired: 2 in, 2 out]
                n267 = property on="Aquire" class="Bool (strict)"("DisabledEnum"=T1."Enabled" ("禁用")) -> ()  [unwired: 2 in, 2 out]
              }
            }
          }
        }
      }
    }
    frame #2 {
      n268 = Release Queue(queue=w409) -> ()  [unwired: 2 in, 3 out]
      n269 = Release Queue(queue=w411) -> ()  [unwired: 2 in, 3 out]
      n270 = Release Queue(queue=w410) -> ()  [unwired: 2 in, 3 out]
    }
  }
